vi "CAEN_STRING_DATA (SubVI).vi"(10 "Value":dbl[](array[numeric]), 11 "Value 2":dbl[](array[numeric])) -> (3 "String":string)   [LabVIEW 2020]
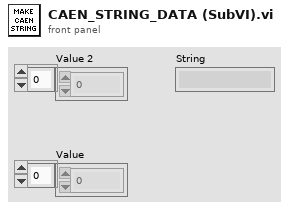
[diagram p1: front panel]
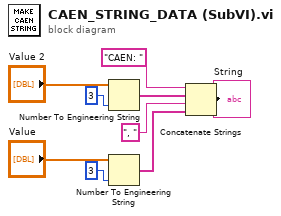
[diagram p0: block diagram]
diagram:
  n1 = Number To Engineering String(2:i16 3 ("precision (6)"), 4:"Value 2") -> (0:w1:string[])  [unwired: 2 in]
  n2 = Number To Engineering String(2:i16 3 ("precision (6)"), 4:"Value") -> (0:w3:string[])  [unwired: 2 in]
  n3 = Concatenate Strings("CAEN: ", w1, ", ", w3) -> (→"String":string)
